vi "construct.vi"(8 "error in (no error)":errorcluster, 9 "configuration name":string, 10 "load config file?":bool=TRUE, 11 "DL090324Microscope in":refnum<class "InstrumentDL090324.lvclass">) -> (0 "error out":errorcluster, 3 "DL090324Microscope out":refnum<class "InstrumentDL090324.lvclass">)   [LabVIEW 2010, in "InstrumentDL090324.lvclass"]
uses:
  InstrumentDL090324.lvclass
  GenericInstrument/GenericInstrument/GenericInstrument.lvclass
  LightSource/GenericLightSource/GenericLightSource/GenericLightSource.lvclass
  Detector/GenericDetector/GenericDetector/GenericDetector.lvclass
  InstrumentDL090324.lvclass/InstrumentDL090324.ctl
  common/classes/GenericComponent/GenericComponent/GenericComponent.lvclass
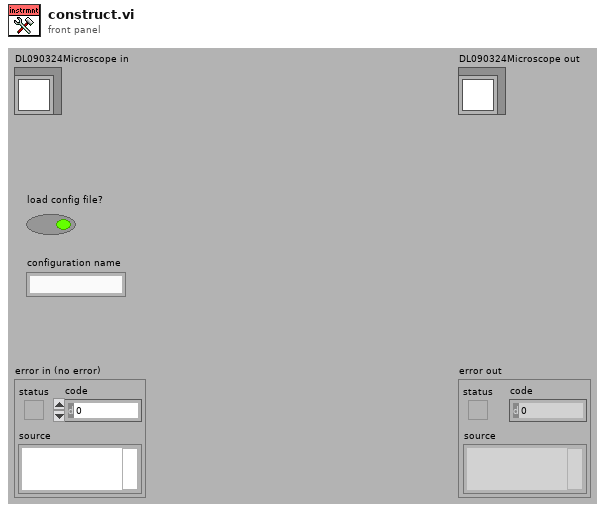
[diagram p1: front panel]
types:
  T1 = typedef "plugin_specification.ctl" = cluster{"class path":string, "configuration":string, "label":string, "settings name":string}
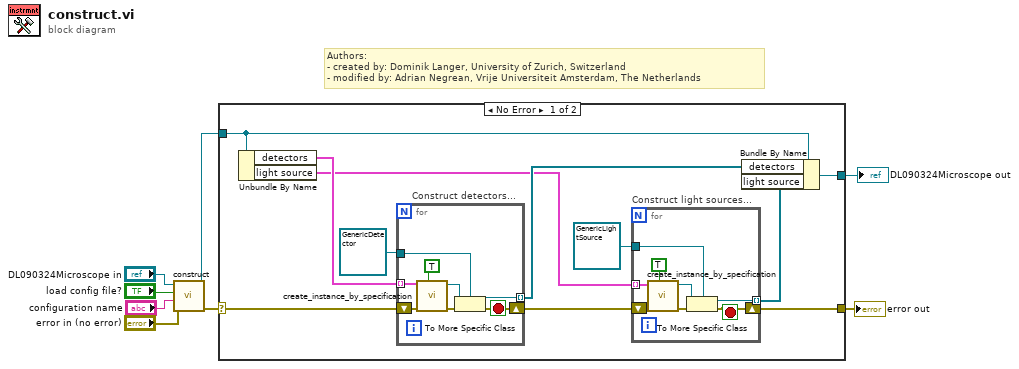
[diagram p0: block diagram]
diagram:
  # "Authors: \n- created by: Dominik Langer, University of Zurich, Switzerland\n- modified by: Adrian Negrean, Vrije Universiteit Amsterdam, The Netherlands"
  n1 = call-parent "construct.vi"("error in (no error)"="error in (no error)", "configuration name"="configuration name", "load config file?"="load config file?", "GenericPlugin in"="DL090324Microscope in") -> ("error out"=w4:errorcluster, "GenericPlugin out"=w3:refnum<class "InstrumentDL090324.lvclass">)  [unwired: 6 out]
  n2 = case shown="No Error" w4 {
    selector: w4 -> [w14 w36]
    tunnel: w3 -> [w15 w37]
    tunnel: [w11 w36] -> w2
    tunnel: [w19 w37] -> w1
    frame No Error {
      n3 = Unbundle By Name(w15) -> ("detectors"=w17:T1[], "light source"=w13:T1[])
      n4 = for "Construct detectors..." {
        tunnel: w17 -> [w34] mode=indexing
        shift-right: [w28] -> w10
        shift-left: w14 -> [w31]
        tunnel: refnum<class "GenericDetector.lvclass"> refnum ("GenericDetector.lvclass") -> [w35]
        tunnel: [w33] -> w16 mode=indexing
        stop <- w28 stop-if-true
        n5 = call "create_instance_by_specification.vi"("call constructor?"=TRUE, "error in (no error)"=w31, "component specification"=w34) -> ("error out"=w30:errorcluster, "GenericPlugin out"=w32:refnum<class "GenericComponent.lvclass">)  [unwired: 6 in, 1 out]
        n6 = To More Specific Class(target class=w35, reference=w32, error in=w30) -> (specific class reference=w33:refnum<class "GenericDetector.lvclass">, error out=w28:errorcluster)
      }
      n7 = for "Construct light sources..." {
        tunnel: w13 -> [w27] mode=indexing
        tunnel: [w23] -> w9 mode=indexing
        shift-right: [w20] -> w11
        shift-left: w10 -> [w26]
        tunnel: refnum<class "GenericLightSource.lvclass"> refnum ("GenericLightSource.lvclass") -> [w21]
        stop <- w20 stop-if-true
        n8 = call "create_instance_by_specification.vi"("call constructor?"=TRUE, "error in (no error)"=w26, "component specification"=w27) -> ("error out"=w25:errorcluster, "GenericPlugin out"=w24:refnum<class "GenericComponent.lvclass">)  [unwired: 6 in, 1 out]
        n9 = To More Specific Class(target class=w21, reference=w24, error in=w25) -> (specific class reference=w23:refnum<class "GenericLightSource.lvclass">, error out=w20:errorcluster)
      }
      n10 = Bundle By Name(cluster=w15, "detectors"=w16, "light source"=w9) -> (w19:refnum<class "InstrumentDL090324.lvclass">)
    }
    frame Error {
    }
  }
  "error out" <- w2
  "DL090324Microscope out" <- w1
